vi "SetLatch.vi"(9 "latch":bool, 10 "latch value":string, 11 "condition in":T1) -> (3 "condition out":T1)   [LabVIEW 2017, in "Trigger.lvlib"]
uses:
  <vilib>/addons/InsightCM/Devices/Shared/Common/Trigger/Trigger.lvlib
  <vilib>/addons/InsightCM/Devices/Shared/Common/Trigger/controls/TriggerCondition.ctl
  <vilib>/addons/InsightCM/MessageBus/Base/controls/Condition.ctl
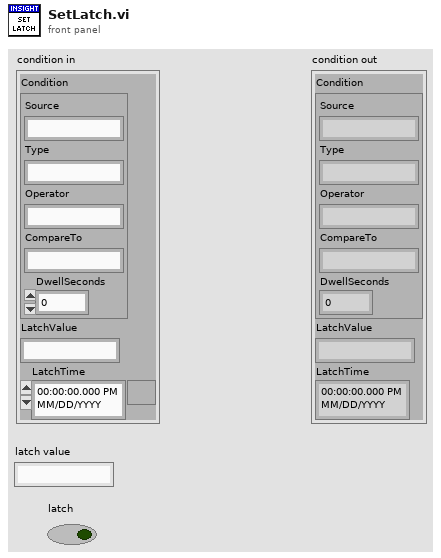
[diagram p1: front panel]
types:
  T1 = typedef "Trigger.lvlib/TriggerCondition.ctl" = cluster{"Condition":T2, "LatchValue":string, "LatchTime":timestamp}
  T2 = typedef "Condition.ctl" = cluster{"Source":string, "Type":string, "Operator":string, "CompareTo":string, "DwellSeconds":dbl}
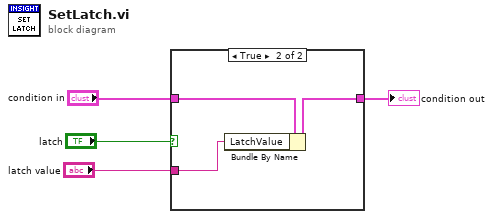
[diagram p0: block diagram]
diagram:
  n1 = case shown="True" "latch" {
    tunnel: "condition in" -> [w5 w8]
    tunnel: [w5 w7] -> w3
    tunnel: "latch value" -> [_ w6]
    frame False {
    }
    frame True {
      n2 = Bundle By Name(cluster=w8, "LatchValue"=w6) -> (w7:T1)
    }
  }
  "condition out" <- w3
